vi "dosya kaydetme.vi"() -> ()   [LabVIEW 2015]
uses:
  <vilib>/Utility/file.llb/Write Delimited Spreadsheet (DBL).vi
  <vilib>/Utility/file.llb/Read Delimited Spreadsheet (DBL).vi
panel:
  in  "file path (dialog if empty)":path
  out "Waveform Graph":dbl[][](graph)
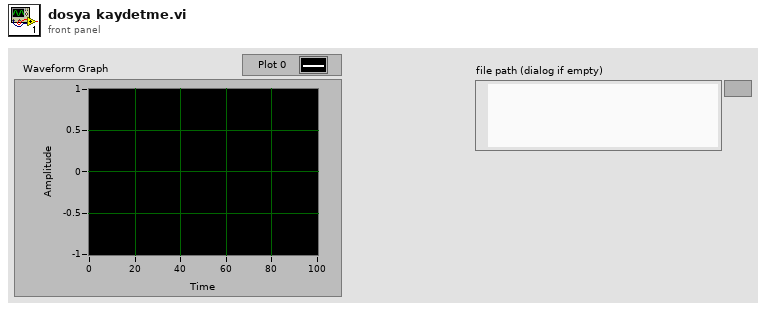
[diagram p1: front panel]
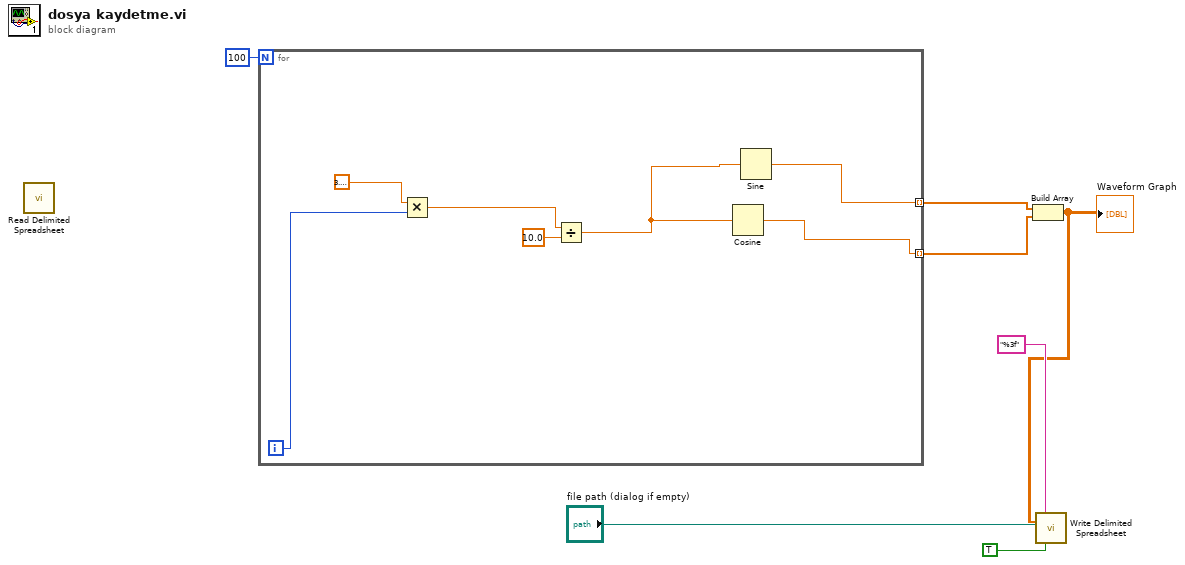
[diagram p0: block diagram]
diagram:
  n1 = call-poly <vilib>:"Read Delimited Spreadsheet.vi"() -> ()  [unwired: 10 in, 6 out]
  n2 = for {
    N: 100 -> [_]
    tunnel: [w9] -> w6 mode=indexing
    tunnel: [w8] -> w5 mode=indexing
    i -> [w12]
    n3 = Multiply(x=3.141592653589793, y=w12) -> (x*y=w11:dbl)
    n4 = Divide(x=w11, y=10.0) -> (x/y=w10:dbl)
    n5 = Cosine(x=w10) -> (cos(x)=w8:dbl)
    n6 = Sine(x=w10) -> (sin(x)=w9:dbl)
  }
  n7 = Build Array(w6, w5) -> (w1:dbl[][])
  "Waveform Graph" <- w1
  n8 = call-poly <vilib>:"Write Delimited Spreadsheet.vi"("file path (dialog if empty)"="file path (dialog if empty)", "format (%.3f)"="%3f", "2D data"=w1, "transpose? (F)"=TRUE) -> ()  [unwired: 10 in, 2 out]
